vi "avToStringScalarAv.vi"(1 "attribute value":T2={"device name"="", "attribute name"="", "quality value"=0, "quality string"="", "timestamp"=0.0, "dim. x"=0, "dim. y"=0, "value"=[], "error code"=0, "error stack"=[], "data type"=36}) -> (0 "av":T1)   [LabVIEW 2014, in "tango.lvlib"]
uses:
  tango.lvlib
  base/toStringScalar.vi
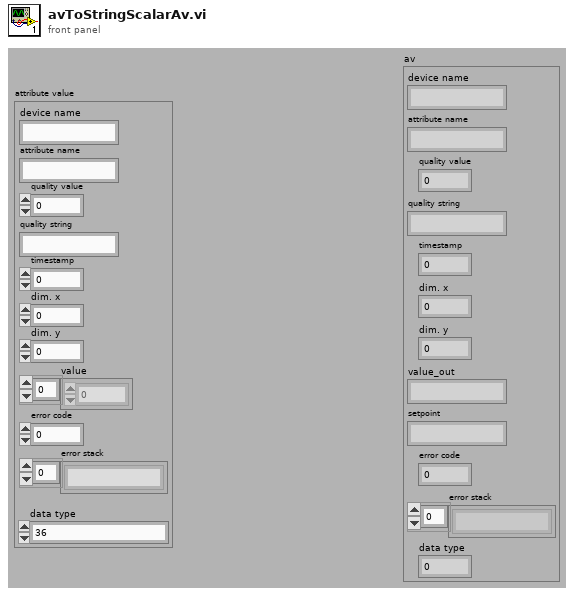
[diagram p1: front panel]
types:
  T1 = cluster{"device name":string, "attribute name":string, "quality value":i16, "quality string":string, "timestamp":dbl, "dim. x":i32, "dim. y":i32, "value_out":string, "setpoint":string, "error code":i32, "error stack":string[], "data type":u16}
  T2 = cluster{"device name":string, "attribute name":string, "quality value":i16, "quality string":string, "timestamp":dbl, "dim. x":i32, "dim. y":i32, "value":u8[], "error code":i32, "error stack":string[], "data type":u16}
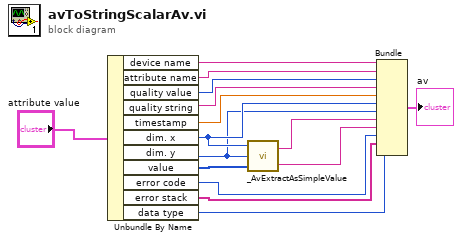
[diagram p0: block diagram]
diagram:
  n1 = Unbundle By Name("attribute value") -> ("device name"=w14:string, "attribute name"=w13:string, "quality value"=w12:i16, "quality string"=w11:string, "timestamp"=w10:dbl, "dim. x"=w9:i32, "dim. y"=w8:i32, "value"=w15:u8[], "error code"=w5:i32, "error stack"=w4:string[], "data type"=w2:u16)
  n2 = call-poly "_AvExtractAsSimpleValue.vi"("value_in"=w15, "dim_y"=w8, "dim_x"=w9) -> ("setpoint"=w6:string, "value_out"=w7:string)
  n3 = Bundle("device name"=w14, "attribute name"=w13, "quality value"=w12, "quality string"=w11, "timestamp"=w10, "dim. x"=w9, "dim. y"=w8, "value_out"=w7, "setpoint"=w6, "error code"=w5, "error stack"=w4, "data type"=w2) -> (→"av":T1)  [unwired: 1 in]
